vi "Exemple.vi"() -> ()   [LabVIEW 2019]
panel:
  in  "LabView Port":u16=4000
  in  "pwd":string="midas"
  out "Numeric Indicator":dbl
  out "String":string
  in  "Exit Button":bool
  in  "Numeric Control U16":u16
  in  "Boolean Button":bool=TRUE
  in  "Numeric Control DBL":dbl
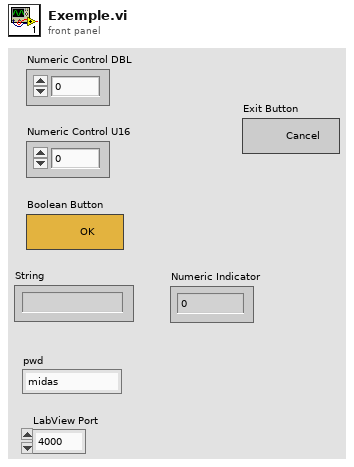
[diagram p1: front panel]
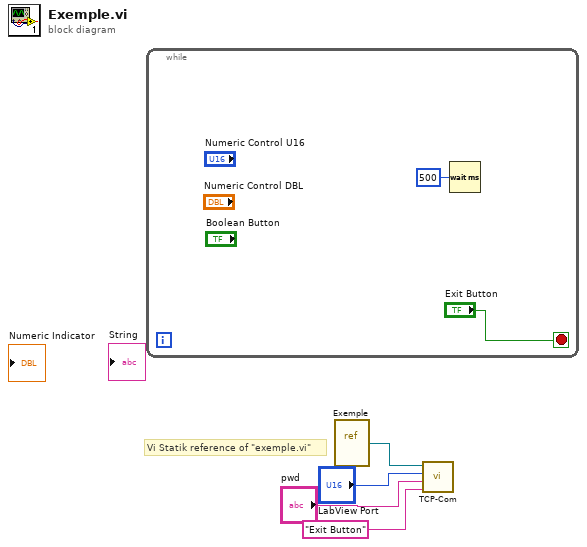
[diagram p0: block diagram]
diagram:
  # "Vi Statik reference of \"exemple.vi\""
  n1 = while {
    stop <- "Exit Button" stop-if-true
    n2 = Wait (ms)(milliseconds to wait=u32 500) -> ()  [unwired: 1 out]
  }
  n3 = vi-ref "Exemple.vi"() -> (w4:refnum<vi>)
  n4 = call "TCP-Com.vi"("Exit Control Label"="Exit Button", "pwd"="pwd", "LabView Port"="LabView Port", "VI Refnum"=w4) -> ()  [unwired: 7 in, 1 out]
